vi "Actor Core.vi"(8 "error in":errorcluster, 11 "Fault Handler in":refnum<class "Fault Handler.lvclass">) -> (0 "error out":errorcluster, 3 "Actor out":refnum<class "Actor.lvclass">)   [LabVIEW 2019, in "Fault Handler.lvlib" / "Fault Handler.lvclass"]
doc: "<b>Bottom Panel</b> actor is an abstraction that provides the actor framework panel size definitions.\n\n<b>Fault Handler</b> This override implements the fault monitor software. \n\n<b> Events </b>\n\n1. Waits for a fault event to be triggered (Events generated by <b>Engine:Check For Errors</b> called consistently through the software. When an event is triggered, the software calls <b> Process Warning</b> or <b>Process Error</b> based on the Status bit of the error cluster.\n\n2. Monitors the Automation Reference Event (generated by <b>Engine:Send Automation Reference</b>) if a reference is provided, the software stores the reference in to private data so the fault handler has the capability of generating faults on the automated software.\n\n<b>User Events</b>\n\n1. After warnings and faults are dealt with, the fault records are cleared by operator intervention clicking clear alarms or clear warnings. \n\n2. The operator can also trigger a hide faults panel action which calls <b>Send Toggle Display</b> routine"
uses:
  Project/Fault Handler.lvclass
  C:/Users/Public/Documents/Development/builds/Engine/Engine.lvlibp/Project/Engine.lvclass
  builds/Engine/Actor Framework.lvlibp/1abvi3w/vi.lib/ActorFramework/Actor/Actor.lvclass
  Project/Fault Handler.lvclass/Fault Handler.ctl
  Accessors/Write Active Alarms.vi
  Accessors/Write Active Warnings.vi
  Accessors/Write Alarm Log.vi
  Accessors/Write Warning Log.vi
  Accessors/Write Faults Tab.vi
  builds/Engine/Engine.lvlibp/Accessors/Write VI_Ref.vi
  builds/Base Software/Panels/Bottom Panel.lvlibp/Project/Bottom.lvclass
panel:
  in  "Hide Faults":bool
  in  "Clear Alarms":bool
  in  "Clear Warnings":bool
  in  "Faults Tab":enum32{"Alarms", "Warnings"}(tab)
  out "Alarm Log":string
  out "Active Alarms":i32(listbox)
  out "Active Warnings":i32(listbox)
  out "Warnings Log":string
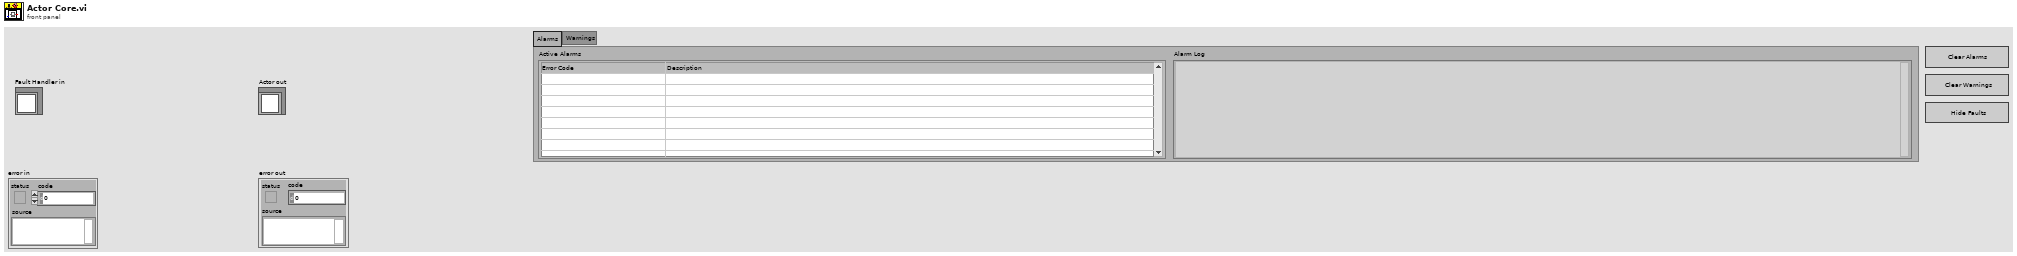
[diagram p1: front panel]
types:
  T1 = cluster{"Pnl Actor":refnum<event-registration>, "Event Registration Refnum":refnum<event-registration>}
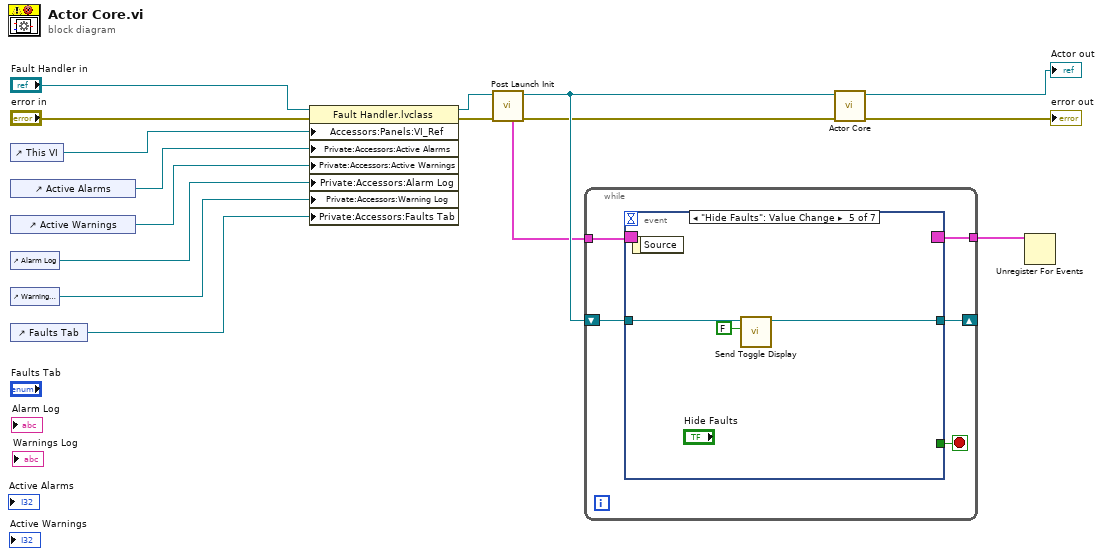
[diagram p0: block diagram]
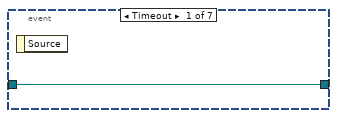
[diagram p2: hidden frame]
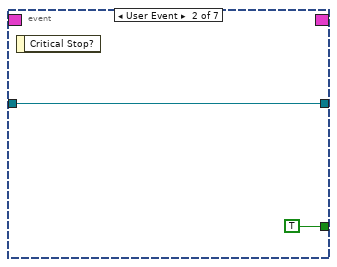
[diagram p3: hidden frame]
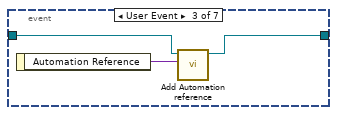
[diagram p4: hidden frame]
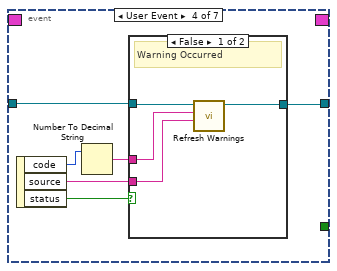
[diagram p5: hidden frame]
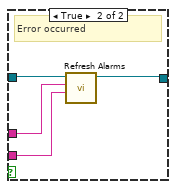
[diagram p6: hidden frame]
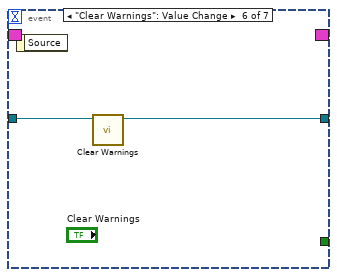
[diagram p7: hidden frame]
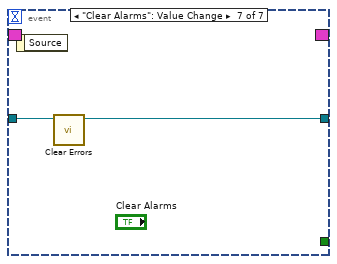
[diagram p8: hidden frame]
diagram:
  n1 = control-ref of="This VI"() -> (w12:refnum<vi>)
  n2 = control-ref of="Active Alarms"() -> (w5:refnum<vi>)
  n3 = control-ref of="Active Warnings"() -> (w4:refnum<vi>)
  n4 = control-ref of="Alarm Log"() -> (w3:refnum<vi>)
  n5 = control-ref of="Warnings Log"() -> (w2:refnum<vi>)
  n6 = control-ref of="Faults Tab"() -> (w1:refnum<vi>)
  n7 = property class="Fault Handler.lvclass"(reference="Fault Handler in", error in="error in", "Accessors:Panels:VI_Ref"=w12, "Private:Accessors:Active Alarms"=w5, "Private:Accessors:Active Warnings"=w4, "Private:Accessors:Alarm Log"=w3, "Private:Accessors:Warning Log"=w2, "Private:Accessors:Faults Tab"=w1) -> (reference out=w9:refnum<class "Fault Handler.lvclass">, error out=w10:errorcluster)
  n8 = call "Post Launch Init.vi"("error in"=w10, "Fault Handler in"=w9) -> ("error out"=w7:errorcluster, "Fault Handler out"=w8:refnum<class "Fault Handler.lvclass">, "Events"=w6:T1)  [unwired: 7 in]
  n9 = while {
    tunnel: w6 -> [w21]
    tunnel: [w20] -> w11
    shift-right: [w17] -> _
    shift-left: w8 -> [w18]
    stop <- w19 stop-if-true
    n10 = event shown="[4] \"Hide Faults\": Value Change" {
      selector: w21 -> [_ _ _ _ _ _ _]
      dyn-events: [_ _ _ _ _ _ _] -> w20
      timeout: _ -> [_ _ _ _ _ _ _]
      tunnel: [_ TRUE _ _ _ _ _] -> w19
      tunnel: w18 -> [w22 w23 w27 w32 w44 w46 w48]
      tunnel: [w22 w23 w25 w28 w42 w45 w47] -> w17
      event Timeout {
        n11 = event-data() -> ()  [unwired: 1 in, 1 out]
      }
      event User Event {
        n12 = event-data() -> ()  [unwired: 1 in, 1 out]
      }
      event User Event {
        n13 = event-data() -> ("Automation Reference"=w26:variant)  [unwired: 1 in]
        n14 = call "Add Automation reference.vi"("Automation"=w26, "Fault Handler in"=w27) -> ("Fault Handler out"=w25:refnum<class "Fault Handler.lvclass">)  [unwired: 8 in, 1 out]
      }
      event User Event {
        n15 = event-data() -> ("code"=w29:i32, "source"=w33:string, "status"=w31:bool)  [unwired: 1 in]
        n16 = Number To Decimal String(number=w29) -> (decimal integer string=w30:string)  [unwired: 1 in]
        n17 = case shown="False" w31 {
          tunnel: w33 -> [w35 w40]
          tunnel: w32 -> [w37 w41]
          tunnel: w30 -> [w36 w39]
          tunnel: [w34 w38] -> w28
          frame False {
            # "Warning Occurred"
            n18 = call "Refresh Warnings.vi"("Source"=w35, "Code"=w36, "Fault Handler in"=w37) -> ("Fault Handler out"=w34:refnum<class "Fault Handler.lvclass">)  [unwired: 7 in, 1 out]
          }
          frame True {
            # "Error occurred"
            n19 = call "Refresh Alarms.vi"("Source"=w40, "Code"=w39, "Fault Handler in"=w41) -> ("Fault Handler out"=w38:refnum<class "Fault Handler.lvclass">)  [unwired: 7 in, 1 out]
          }
        }
      }
      event "Hide Faults": Value Change {
        n20 = event-data() -> ()  [unwired: 1 in, 1 out]
        n21 = call "Send Toggle Display.vi"("Show"=FALSE, "Fault Handler in"=w44) -> ("Fault Handler out"=w42:refnum<class "Fault Handler.lvclass">)  [unwired: 8 in, 1 out]
      }
      event "Clear Warnings": Value Change {
        n22 = event-data() -> ()  [unwired: 1 in, 1 out]
        n23 = call "Clear Warnings.vi"("Fault Handler in"=w46) -> ("Fault Handler out"=w45:refnum<class "Fault Handler.lvclass">)  [unwired: 9 in, 1 out]
      }
      event "Clear Alarms": Value Change {
        n24 = event-data() -> ()  [unwired: 1 in, 1 out]
        n25 = call "Clear Errors.vi"("Fault Handler in"=w48) -> ("Fault Handler out"=w47:refnum<class "Fault Handler.lvclass">)  [unwired: 9 in, 1 out]
      }
    }
  }
  n26 = call-parent "Actor Core.vi"("error in"=w7, "Bottom in"=w8) -> ("error out"=→"error out":errorcluster, "Actor out"=→"Actor out":refnum<class "Actor.lvclass">)  [unwired: 8 in]
  n27 = Unregister For Events(event registration refnum=w11) -> ()  [unwired: 1 in, 1 out]
